vi "SMR_LabVIEW_V8.vi"() -> ()   [LabVIEW 2025]
uses:
  <vilib>/DAQmx/write.llb/DAQmx Write (Analog DBL 1Chan 1Samp).vi
  <vilib>/DAQmx/read.llb/DAQmx Read (Analog 1D DBL NChan 1Samp).vi
  <vilib>/DAQmx/read.llb/DAQmx Read (Analog 2D DBL NChan NSamp).vi
  <vilib>/Analysis/baseanly.llb/Mean (DBL).vi
  <vilib>/DAQmx/create/channels.llb/DAQmx Create Channel (AI-Temperature-Thermocouple).vi
  <vilib>/DAQmx/create/channels.llb/DAQmx Create Channel (AI-Voltage-Basic).vi
  <vilib>/DAQmx/create/channels.llb/DAQmx Create Channel (AO-Voltage-Basic).vi
  <vilib>/DAQmx/miscellaneous.llb/DAQmx Fill In Error Info.vi
  <vilib>/DAQmx/configure/timing.llb/DAQmx Timing (Sample Clock).vi
  <vilib>/addons/control/pid/pid.llb/PID (DBL).vi
  <vilib>/measure/maspectr.llb/FFT Power Spectrum and PSD for 1 Chan.vi
  <vilib>/measure/matone.llb/Extract Single Tone Information 1 Chan.vi
  <vilib>/addons/control/pid/NI_PID_pid.lvlib
  <vilib>/Analysis/NI_AALBase.lvlib
  <vilib>/ptbypt/NI_PtbyPt.lvlib
  <vilib>/measure/NI_MAPro.lvlib
panel:
  out "Time in Steady State (s)":dbl
  in  "Steady-State Dwell (s)":dbl
  out "Main Loop Flow (GPM)":dbl
  out "FM Amplitude":dbl
  out "FM Frequency":dbl
  out "Spectrum":cluster{"f0":dbl, "df":dbl, "magnitude":dbl[]}(graph)
  out "Raw Signal":waveform(dbl)(graph)
  out "Smoothed HX Flow (GPM)":dbl
  out "Flow History":dbl(graph)
  out "HX Flow (GPM)":dbl
  out "Voltage Across Rod (V)":dbl format="%0.2f"
  out "Current Run Folder":path
  in  "Log Root Folder":path=path "C:/Users/LocalUser/Documents/GitHub/thermal-loop/resources/v0.1.1/data/001"
  out "Raw NI9201 \nVoltage Display":T1
  in  "Loop Period (ms)":dbl=1000.0
  in  "Stop":bool
  out "Auto Steady State Threshold (deg C/min)":dbl
  out "Max dT/dt (deg C/min)":dbl
  out "Temp Change Rate (deg C/min)":dbl
  out "5-Min Baseline Complete":bool
  out "Rate Window Ready":bool
  out "Steady State":bool
  in  "Voltage Limit (V)":dbl=10.0
  in  "Temperature Limit (C)":dbl=50.0
  in  "Pressure Limit (psi)":dbl=15.0
  out "Max Voltage":bool
  out "Max Temperature":bool
  out "Max Pressure":bool
  out "Heat Exchanger Pressure History":dbl(graph)
  out "Main Loop Pressure History":T2(graph)
  out "Overall Avg Pressure (psi)":dbl
  out "Heat Exchanger Pressure P6 (psi)":dbl
  out "Main Loop Avg Pressure (psi)":dbl
  out "Pressure Display":T3
  out "Overall Pressure History":T4(graph)
  out "Max Loop Pressure (psi)":dbl
  out "Heat Exchanger Temperature History":cluster{"Waveform":dbl, "Waveform":dbl}(graph)
  out "Main Loop Temeperature History":T5(graph)
  out "Heat Exchanger Avg Temp (deg C)":dbl
  out "Temperature Display":T6
  out "Overall Temperature History":T7(graph)
  out "Overall Avg Temp (deg C)":dbl
  out "Max Loop Temp (deg C)":dbl
  out "Final P-Valve Voltage (V)":dbl
  out "PID Trim Voltage (V)":dbl
  in  "PID Temp Setpoint (deg C)":dbl
  in  "Auto PID Enable":bool
  in  "Manual P-Valve Voltage (V)":dbl min=0.0 max=10.0
  out "Main Loop Avg Temp (deg C)":dbl
  # "Heat Exchanger Flow"
  # "Control/Troubleshoot"
  # "Steady State"
  # "Emergency Indicators"
  # "Pressure"
  # "Temperature"
  # "Proportional Valve Control"
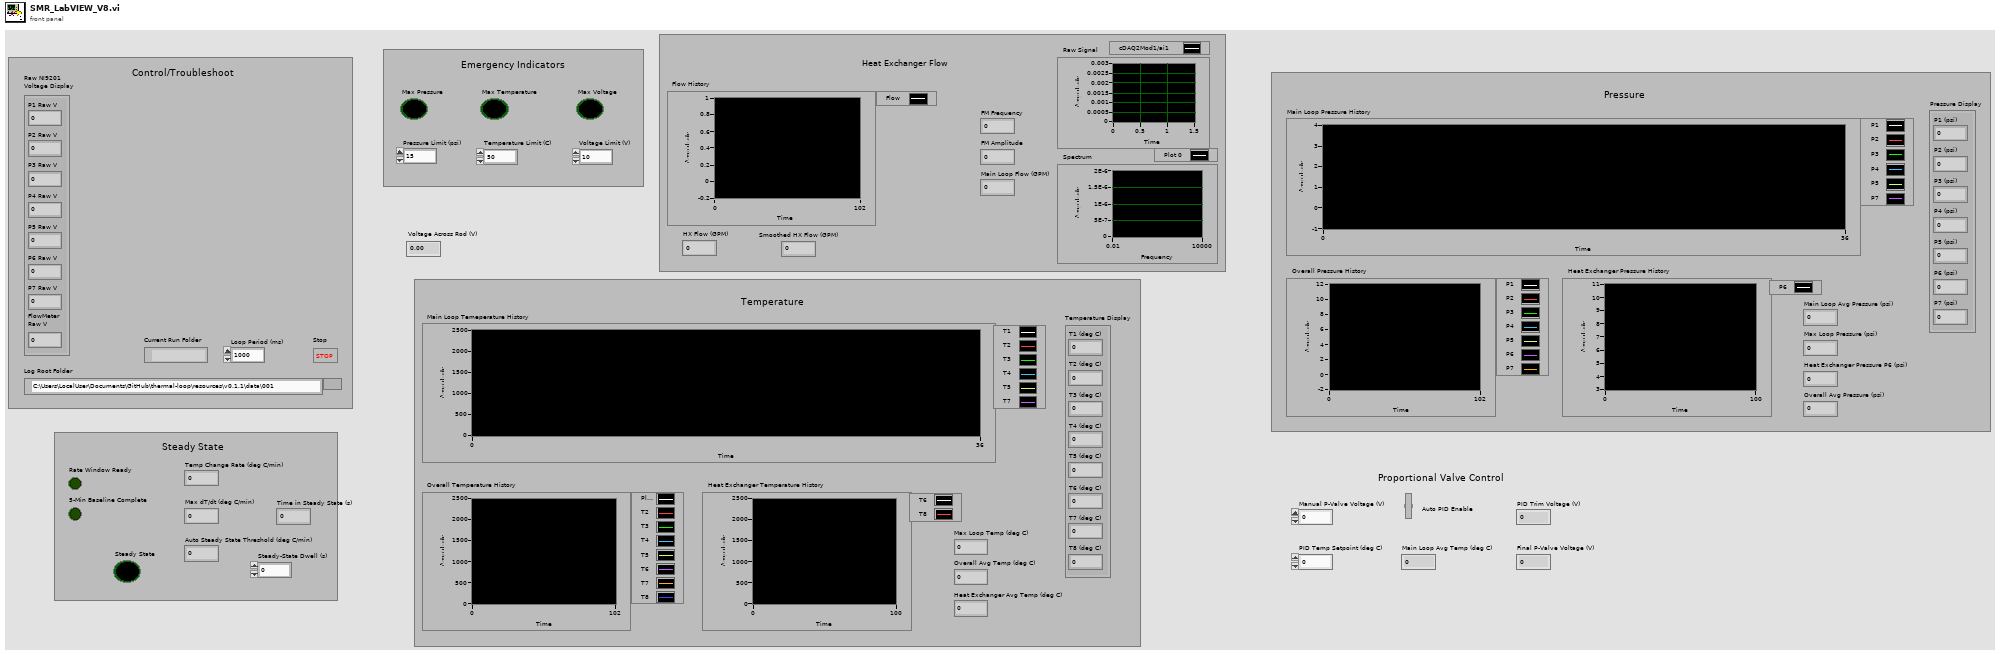
[diagram p1: front panel]
types:
  T1 = cluster{"P1 Raw V":dbl, "P2 Raw V":dbl, "P3 Raw V":dbl, "P4 Raw V":dbl, "P5 Raw V":dbl, "P6 Raw V":dbl, "P7 Raw V":dbl, "FlowMeter\nRaw V":dbl}
  T2 = cluster{"P1":dbl, "P2":dbl, "P3":dbl, "P4":dbl, "P5":dbl, "P7":dbl}
  T3 = cluster{"P1 (psi)":dbl, "P2 (psi)":dbl, "P3 (psi)":dbl, "P4 (psi)":dbl, "P5 (psi)":dbl, "P6 (psi)":dbl, "P7 (psi)":dbl}
  T4 = cluster{"P1":dbl, "P2":dbl, "P3":dbl, "P4":dbl, "P5":dbl, "P6":dbl, "P7":dbl}
  T5 = cluster{"Waveform":dbl, "Waveform":dbl, "Waveform":dbl, "Waveform":dbl, "Waveform":dbl, "Waveform":dbl}
  T6 = cluster{"T1 (deg C)":dbl, "T2 (deg C)":dbl, "T3 (deg C)":dbl, "T4 (deg C)":dbl, "T5 (deg C)":dbl, "T6 (deg C)":dbl, "T7 (deg C)":dbl, "T8 (deg C)":dbl}
  T7 = cluster{"Waveform":dbl, "Waveform":dbl, "Waveform":dbl, "Waveform":dbl, "Waveform":dbl, "Waveform":dbl, "Waveform":dbl, "Waveform":dbl}
  T8 = enum16{"open", "replace", "create", "open or create", "replace or create", "replace or create with confirmation"}
  T9 = cluster{"proportional gain (Kc)":dbl, "integral time (Ti, min)":dbl, "derivative time (Td, min)":dbl}
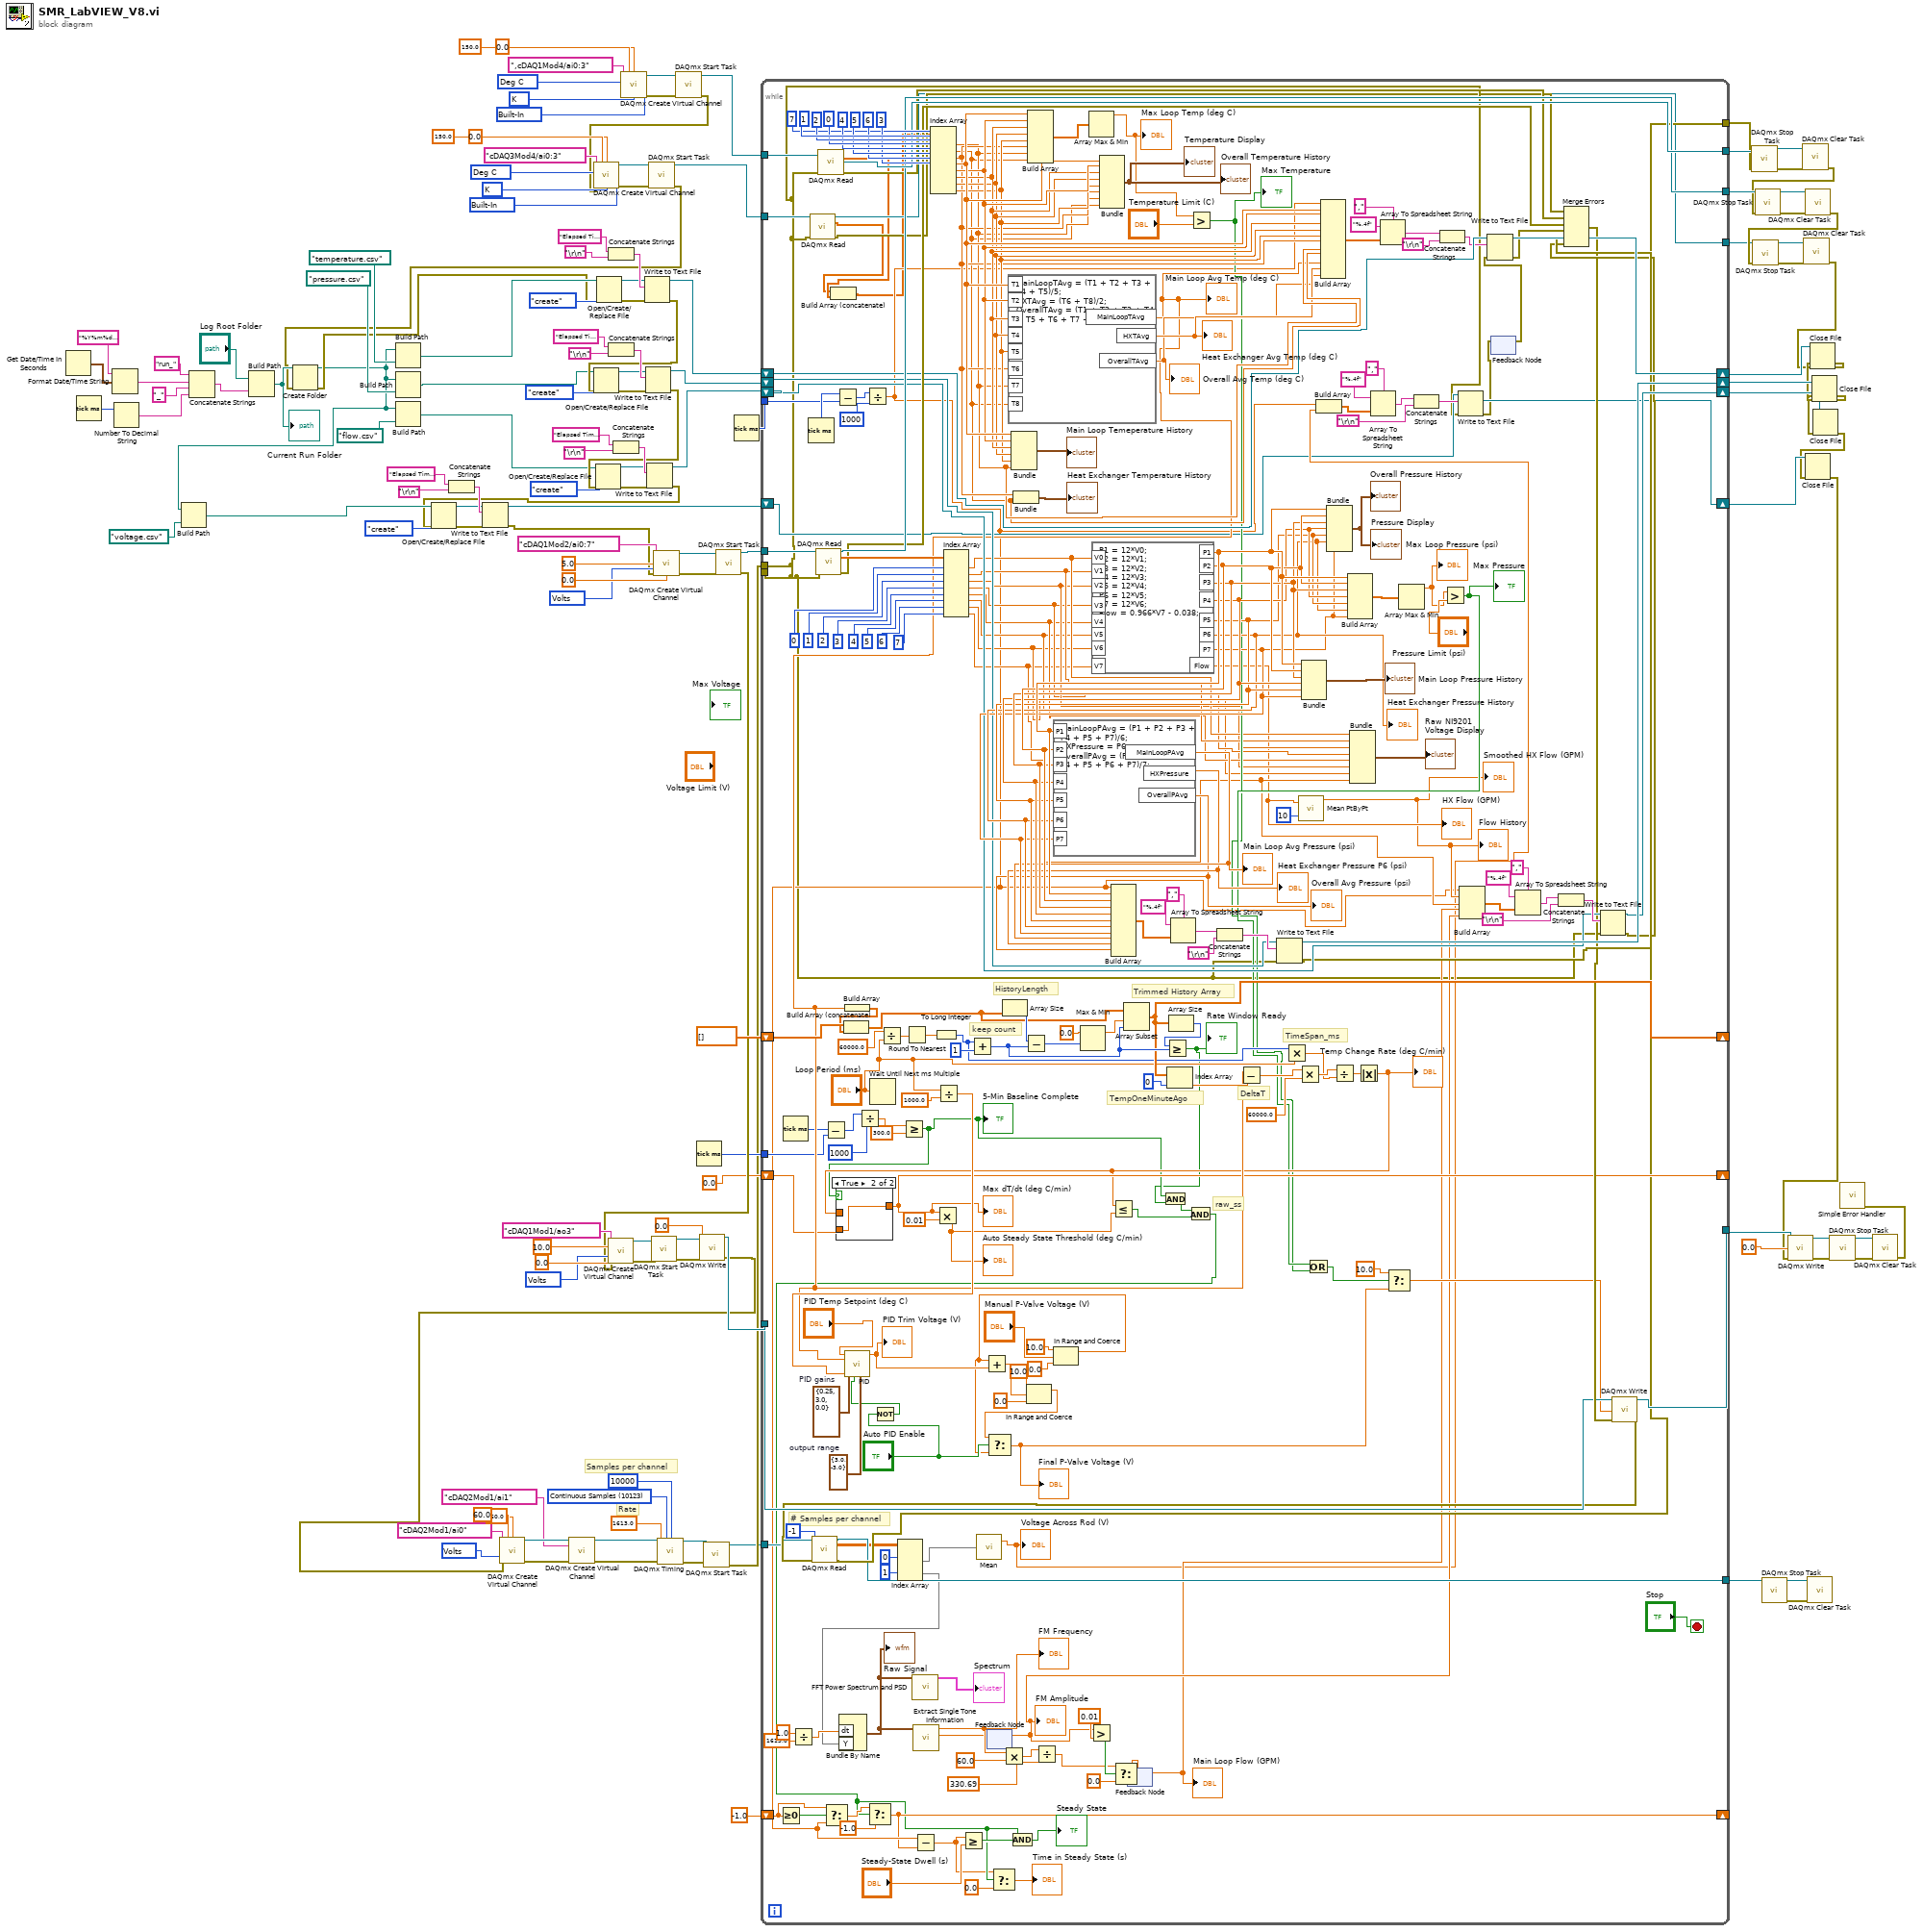
[diagram p0: block diagram]
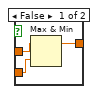
[diagram p2: hidden frame]
diagram:
  w12 = 10200 items=["Built-In"=10200, "Constant Value"=10116, "Channel"=10113] ("cjc source")
  w13 = 10073 items=["J"=10072, "K"=10073, "N"=10077, "R"=10082, "S"=10085, "T"=10086, "B"=10047, "E"=10055] ("thermocouple type")
  w14 = 10143 items=["Deg C"=10143, "Deg F"=10144, "Kelvins"=10325, "Deg R"=10145, "From Custom Scale"=10065] ("units")
  w47 = 10123 items=["Finite Samples"=10178, "Continuous Samples"=10123, "Hardware Timed Single Point"=12522] ("sample mode")
  w49 = 10348 items=["Volts"=10348, "From Custom Scale"=10065] ("units")
  w69 = 10348 items=["Volts"=10348, "From Custom Scale"=10065] ("units")
  w131 = 10200 items=["Built-In"=10200, "Constant Value"=10116, "Channel"=10113] ("cjc source")
  w132 = 10073 items=["J"=10072, "K"=10073, "N"=10077, "R"=10082, "S"=10085, "T"=10086, "B"=10047, "E"=10055] ("thermocouple type")
  w133 = 10143 items=["Deg C"=10143, "Deg F"=10144, "Kelvins"=10325, "Deg R"=10145, "From Custom Scale"=10065] ("units")
  w140 = 10348 items=["Volts"=10348, "From Custom Scale"=10065] ("units")
  # "Samples per channel"
  # "Rate"
  n1 = Get Date/Time In Seconds() -> (seconds since 1Jan1904=w90:timestamp)
  n2 = Tick Count (ms)() -> (millisecond timer value=w88:u32)
  n3 = Format Date/Time String(time format string (%c)="%Y%m%d_%H%M%S", seconds (now)=w90) -> (date/time string=w85:string)  [unwired: 1 in]
  n4 = Number To Decimal String(number=w88) -> (decimal integer string=w86:string)  [unwired: 1 in]
  n5 = Concatenate Strings("run_" ("string"), w85, "_" ("string"), w86) -> (w82:string)
  n6 = Build Path(base path="Log Root Folder", name or relative path=w82) -> (appended path=w81:path)
  "Current Run Folder" <- w81
  n7 = Concatenate Strings("Elapsed Time (s), Rod voltage (V)", "\r\n") -> (w31:string)
  n8 = Concatenate Strings("Elapsed Time (s),T1 (deg C),T2 (deg C),T3 (deg C),T4 (deg C),T5 (deg C),T6 (deg C),T7 (deg C),T8 (deg C),Main Loop Avg Temp (deg C),HX Avg Temp (deg C),Overall Avg Temp (deg C)", "\r\n") -> (w114:string)
  n9 = Concatenate Strings("Elapsed Time (s),P1 (psi),P2 (psi),P3 (psi),P4 (psi),P5 (psi),P6 (psi),P7 (psi),Main Loop Avg Pressure (psi),HX Pressure (psi),Overall Avg Pressure (psi)", "\r\n") -> (w112:string)
  n10 = Concatenate Strings("Elapsed Time (s),Heat Exchanger Flow (GPM),Flow Raw Voltage (V), Main Loop Flow (GPM), Flow Signal Amplitude (V)", "\r\n") -> (w108:string)
  n11 = call-poly <vilib>:"DAQmx Create Virtual Channel.vi"("maximum value"=150.0, "minimum value"=0.0, "physical channels"=tag ",cDAQ1Mod4/ai0:3", "cjc source"=w131, "units"=w133, "thermocouple type"=w132) -> ("task out"=w130:refnum<k21>, "error out"=w129:errorcluster)  [unwired: 8 in]
  n12 = call <vilib>:"DAQmx Start Task.vi"("task/channels in"=w130, "error in"=w129) -> ("task out"=w128:refnum<k21>, "error out"=w8:errorcluster)  [unwired: 12 in]
  n13 = call-poly <vilib>:"DAQmx Create Virtual Channel.vi"("maximum value"=150.0, "minimum value"=0.0, "physical channels"=tag "cDAQ3Mod4/ai0:3", "cjc source"=w12, "units"=w14, "error in"=w8, "thermocouple type"=w13) -> ("task out"=w11:refnum<k21>, "error out"=w10:errorcluster)  [unwired: 7 in]
  n14 = call <vilib>:"DAQmx Start Task.vi"("task/channels in"=w11, "error in"=w10) -> ("task out"=w6:refnum<k21>, "error out"=w7:errorcluster)  [unwired: 12 in]
  n15 = Create Folder(path (use dialog)=w81, error in=w7) -> (created path=w25:path, error out=w74:errorcluster)  [unwired: 1 in, 1 out]
  n16 = Build Path(base path=w25, name or relative path=path "voltage.csv") -> (appended path=w26:path)
  n17 = Build Path(base path=w25, name or relative path=path "temperature.csv") -> (appended path=w80:path)
  n18 = Build Path(base path=w25, name or relative path=path "pressure.csv") -> (appended path=w79:path)
  n19 = Build Path(base path=w25, name or relative path=path "flow.csv") -> (appended path=w78:path)
  n20 = Open/Create/Replace File(file path (use dialog)=w80, error in=w74, operation (0:open)=T8."create") -> (refnum out=w113:refnum<file>, error out=w97:errorcluster)  [unwired: 3 in, 1 out]
  n21 = Write to Text File(file (use dialog)=w113, text=w114, error in=w97) -> (refnum out=w104:refnum<file>, error out=w96:errorcluster)  [unwired: 1 in, 1 out]
  n22 = Open/Create/Replace File(file path (use dialog)=w79, error in=w96, operation (0:open)=T8."create") -> (refnum out=w111:refnum<file>, error out=w95:errorcluster)  [unwired: 3 in, 1 out]
  n23 = Write to Text File(file (use dialog)=w111, text=w112, error in=w95) -> (refnum out=w103:refnum<file>, error out=w94:errorcluster)  [unwired: 1 in, 1 out]
  n24 = Open/Create/Replace File(file path (use dialog)=w78, error in=w94, operation (0:open)=T8."create") -> (refnum out=w107:refnum<file>, error out=w93:errorcluster)  [unwired: 3 in, 1 out]
  n25 = Write to Text File(file (use dialog)=w107, text=w108, error in=w93) -> (refnum out=w102:refnum<file>, error out=w23:errorcluster)  [unwired: 1 in, 1 out]
  n26 = Open/Create/Replace File(file path (use dialog)=w26, error in=w23, operation (0:open)=T8."create") -> (refnum out=w30:refnum<file>, error out=w27:errorcluster)  [unwired: 3 in, 1 out]
  n27 = Write to Text File(file (use dialog)=w30, text=w31, error in=w27) -> (refnum out=w21:refnum<file>, error out=w22:errorcluster)  [unwired: 1 in, 1 out]
  n28 = call-poly <vilib>:"DAQmx Create Virtual Channel.vi"("maximum value"=5.0, "minimum value"=0.0, "physical channels"=tag "cDAQ1Mod2/ai0:7", "units"=w140, "error in"=w22) -> ("task out"=w139:refnum<k21>, "error out"=w138:errorcluster)  [unwired: 9 in]
  n29 = Tick Count (ms)() -> (millisecond timer value=w54:u32)
  n30 = call <vilib>:"DAQmx Start Task.vi"("task/channels in"=w139, "error in"=w138) -> ("task out"=w137:refnum<k21>, "error out"=w62:errorcluster)  [unwired: 12 in]
  n31 = call-poly <vilib>:"DAQmx Create Virtual Channel.vi"("maximum value"=10.0, "minimum value"=0.0, "physical channels"=tag "cDAQ1Mod1/ao3", "units"=w69, "error in"=w62) -> ("task out"=w68:refnum<k21>, "error out"=w67:errorcluster)  [unwired: 9 in]
  n32 = call <vilib>:"DAQmx Start Task.vi"("task/channels in"=w68, "error in"=w67) -> ("task out"=w66:refnum<k21>, "error out"=w65:errorcluster)  [unwired: 12 in]
  n33 = call-poly <vilib>:"DAQmx Write.vi"("task/channels in"=w66, "data"=0.0, "error in"=w65) -> ("task out"=w63:refnum<k21>, "error out"=w41:errorcluster)  [unwired: 10 in, 1 out]
  n34 = call-poly <vilib>:"DAQmx Create Virtual Channel.vi"("maximum value"=60.0, "minimum value"=-60.0, "physical channels"=tag "cDAQ2Mod1/ai0", "units"=w49, "error in"=w41) -> ("task out"=w37:refnum<k21>, "error out"=w36:errorcluster)  [unwired: 9 in]
  n35 = call-poly <vilib>:"DAQmx Create Virtual Channel.vi"("task in"=w37, "physical channels"=tag "cDAQ2Mod1/ai1", "error in"=w36) -> ("task out"=w35:refnum<k21>, "error out"=w34:errorcluster)  [unwired: 11 in]
  n36 = call-poly <vilib>:"DAQmx Timing.vi"("task/channels in"=w35, "sample mode"=w47, "samples per channel"=10000, "rate"=1613.0, "error in"=w34) -> ("task out"=w45:refnum<k21>, "error out"=w44:errorcluster)  [unwired: 9 in]
  n37 = call <vilib>:"DAQmx Start Task.vi"("task/channels in"=w45, "error in"=w44) -> ("task out"=w39:refnum<k21>, "error out"=w40:errorcluster)  [unwired: 12 in]
  n38 = Tick Count (ms)() -> (millisecond timer value=w101:u32)
  n39 = while {
    tunnel: w137 -> [w361]
    tunnel: w128 -> [w344]
    tunnel: [w335] -> w127
    tunnel: [w149] -> _
    tunnel: [w334] -> w126
    tunnel: [w210] -> w125
    shift-right: [w311] -> w100
    shift-left: w104 -> [w312]
    shift-right: [w292] -> w99
    shift-left: w103 -> [w293]
    shift-right: [w284] -> w98
    shift-left: w102 -> [w285]
    tunnel: w101 -> [w330]
    shift-right: [w263] -> _
    shift-left: dbl[] [] -> [w276]
    tunnel: w63 -> [w244]
    tunnel: w40 -> [w149]
    tunnel: [w251] -> w60
    tunnel: w54 -> [w233]
    shift-right: [w226] -> _
    shift-left: 0.0 -> [w228]
    tunnel: w39 -> [w209]
    tunnel: [w208] -> w38
    shift-right: [w166] -> w20
    shift-left: w21 -> [w167]
    shift-right: [w158] -> _
    shift-left: -1.0 -> [w162]
    tunnel: w6 -> [w150]
    tunnel: [w147] -> w2
    stop <- "Stop" stop-if-true
    w249 = cluster{"output high":dbl, "output low":dbl} {"output high"=3.0, "output low"=-3.0}  # output range
    w250 = T9 {"proportional gain (Kc)"=0.25, "integral time (Ti, min)"=3.0, "derivative time (Td, min)"=0.0}  # PID gains
    # "raw_ss"
    # "# Samples per channel"
    # "TimeSpan_ms"
    # "DeltaT"
    # "TempOneMinuteAgo"
    # "Trimmed History Array"
    # "HistoryLength"
    # "keep count"
    n40 = Greater Or Equal To 0?(x=w162) -> (x >= 0?=w163:bool)
    n41 = Tick Count (ms)() -> (millisecond timer value=w234:u32)
    n42 = Divide(x=1.0, y=1613.0) -> (x/y=w181:dbl)
    n43 = Tick Count (ms)() -> (millisecond timer value=w331:u32)
    n44 = call-poly <vilib>:"DAQmx Read.vi"("task/channels in"=w150, "error in"=w149) -> ("task out"=w147:refnum<k21>, "data"=w144:dbl[], "error out"=w148:errorcluster)  [unwired: 11 in]
    n45 = call-poly <vilib>:"DAQmx Read.vi"("task/channels in"=w361, "error in"=w149) -> ("task out"=w334:refnum<k21>, "data"=w352:dbl[], "error out"=w332:errorcluster)  [unwired: 11 in]
    n46 = call-poly <vilib>:"DAQmx Read.vi"("task/channels in"=w344, "error in"=w149) -> ("task out"=w335:refnum<k21>, "data"=w145:dbl[], "error out"=w333:errorcluster)  [unwired: 11 in]
    n47 = Subtract(x=w234, y=w233) -> (x-y=w232:u32)
    n48 = Build Array (concatenate)(w144, w145) -> (w146:dbl[])
    n49 = Subtract(x=w331, y=w330) -> (x-y=w329:u32)
    n50 = Divide(x=w232, y=u32 1000) -> (x/y=w230:dbl)
    n51 = Divide(x=w329, y=u32 1000) -> (x/y=w159:dbl)
    n52 = Select(t=w162, s=w163, f=w159) -> (s? t:f=w161:dbl)
    n53 = Wait Until Next ms Multiple(millisecond multiple="Loop Period (ms)") -> ()  [unwired: 1 out]
    n54 = Not(x="Auto PID Enable") -> (.not. x?=w245:bool)
    n55 = Divide(x=60000.0, y="Loop Period (ms)") -> (x/y=w273:dbl)
    n56 = Greater Or Equal?(x=w230, y=300.0) -> (x >= y?=w223:bool)
    "5-Min Baseline Complete" <- w223
    n57 = Round To Nearest(number=w273) -> (nearest integer value=w272:dbl)
    n58 = Index Array(array=w146, index #1=7 ("index"), index #2=1 ("index"), index #3=2 ("index"), index #4=0 ("index"), index #5=4 ("index"), index #6=5 ("index"), index #7=6 ("index"), index #8=3 ("index")) -> (element #1=w321:dbl, element #2=w320:dbl, element #3=w322:dbl, element #4=w327:dbl, element #5=w326:dbl, element #6=w325:dbl, element #7=w324:dbl, element #8=w323:dbl)
    n59 = To Long Integer(number=w272) -> (32bit integer=w260:i32)
    n60 = Divide(x="Loop Period (ms)", y=1000.0) -> (x/y=w246:dbl)
    n61 = Index Array(array=w352, index #1=0 ("index"), index #2=1 ("index"), index #3=2 ("index"), index #4=3 ("index"), index #5=4 ("index"), index #6=5 ("index"), index #7=6 ("index"), index #8=7 ("index")) -> (element #1=w207:dbl, element #2=w206:dbl, element #3=w205:dbl, element #4=w204:dbl, element #5=w203:dbl, element #6=w202:dbl, element #7=w201:dbl, element #8=w200:dbl)
    n62 = Add(x=w260, y=1) -> (x+y=w265:i32)
    n63 = feedback #1() -> (w177:dbl)  [unwired: 1 in]
    "FM Amplitude" <- w177
    n64 = formula code="MainLoopTAvg = (T1 + T2 + T3 + T4 + T5)/5;\nHXTAvg = (T6 + T8)/2;\nOverallTAvg = (T1 + T2 + T3 + T4 + T5 + T6 + T7 + T8)/8;"("T1"=w327, "T2"=w326, "T3"=w325, "T4"=w324, "T5"=w323, "T6"=w322, "T7"=w321, "T8"=w320) -> ("MainLoopTAvg"=w236:dbl, "HXTAvg"=w319:dbl, "OverallTAvg"=w318:dbl)
    "Overall Avg Temp (deg C)" <- w318
    "Main Loop Avg Temp (deg C)" <- w236
    "Heat Exchanger Avg Temp (deg C)" <- w319
    n65 = Build Array(w236) -> (w275:dbl[])
    n66 = Build Array (concatenate)(w276, w275) -> (w267:dbl[])
    n67 = call-poly <vilib>:"PID.vi"("reinitialize? (F)"=w245, "output range"=w249, "dt (s)"=w246, "PID gains"=w250, "process variable"=w236, "setpoint"="PID Temp Setpoint (deg C)") -> ("output"=w243:dbl)  [unwired: 4 in, 1 out]
    "PID Trim Voltage (V)" <- w243
    n68 = Array Size(array=w267) -> (size(s)=w270:i32)
    n69 = Bundle("Waveform"=w327, "Waveform"=w326, "Waveform"=w325, "Waveform"=w324, "Waveform"=w323, "Waveform"=w321) -> (→"Main Loop Temeperature History":T5)  [unwired: 1 in]
    n70 = Bundle("Waveform"=w322, "Waveform"=w320) -> (→"Heat Exchanger Temperature History":cluster{"Waveform":dbl, "Waveform":dbl})  [unwired: 1 in]
    n71 = Subtract(x=w270, y=w265) -> (x-y=w268:i32)
    n72 = Build Array(w327, w326, w325, w324, w323, w322, w321, w320) -> (w362:dbl[])
    n73 = In Range and Coerce(upper limit=10.0, x="Manual P-Valve Voltage (V)", lower limit=0.0) -> (coerced(x)=w238:dbl)  [unwired: 1 out]
    n74 = Add(x=w238, y=w243) -> (x+y=w242:dbl)
    n75 = In Range and Coerce(upper limit=10.0, x=w242, lower limit=0.0) -> (coerced(x)=w237:dbl)  [unwired: 1 out]
    n76 = Select(t=w237, s="Auto PID Enable", f=w238) -> (s? t:f=w215:dbl)
    "Final P-Valve Voltage (V)" <- w215
    n77 = Max & Min(x=0.0, y=w268) -> (max(x,y)=w266:dbl)  [unwired: 1 out]
    n78 = Array Max & Min(array=w362) -> (max value=w278:dbl)  [unwired: 3 out]
    "Max Loop Temp (deg C)" <- w278
    n79 = Greater?(x=w177, y=0.01) -> (0:w185:bool)
    n80 = formula code="P1 = 12*V0;\nP2 = 12*V1;\nP3 = 12*V2;\nP4 = 12*V3;\nP5 = 12*V4;\nP6 = 12*V5; \nP7 = 12*V6;\nFlow = 0.966*V7 - 0.038;"("V0"=w207, "V1"=w206, "V2"=w205, "V3"=w204, "V4"=w203, "V5"=w202, "V6"=w201, "V7"=w200) -> ("P1"=w310:dbl, "P2"=w309:dbl, "P3"=w308:dbl, "P4"=w307:dbl, "P5"=w306:dbl, "P6"=w305:dbl, "P7"=w304:dbl, "Flow"=w199:dbl)
    "HX Flow (GPM)" <- w199
    "Heat Exchanger Pressure History" <- w305
    n81 = formula code="MainLoopPAvg = (P1 + P2 + P3 + P4 + P5 + P7)/6;\nHXPressure = P6;\nOverallPAvg = (P1 + P2 + P3 + P4 + P5 + P6 + P7)/7;"("P1"=w310, "P2"=w309, "P3"=w308, "P4"=w307, "P5"=w306, "P6"=w305, "P7"=w304) -> ("MainLoopPAvg"=w303:dbl, "HXPressure"=w302:dbl, "OverallPAvg"=w301:dbl)
    "Overall Avg Pressure (psi)" <- w301
    "Heat Exchanger Pressure P6 (psi)" <- w302
    "Main Loop Avg Pressure (psi)" <- w303
    n82 = Bundle("Waveform"=w327, "Waveform"=w326, "Waveform"=w325, "Waveform"=w324, "Waveform"=w323, "Waveform"=w322, "Waveform"=w321, "Waveform"=w320) -> (→"Overall Temperature History" →"Temperature Display":T7)  [unwired: 1 in]
    n83 = Build Array(w159, w310, w309, w308, w307, w306, w305, w304, w303, w302, w301) -> (w300:dbl[])
    n84 = Array Subset(array=w267, index=w266, length=w265) -> (w263:dbl[])
    n85 = feedback #2() -> (w175:dbl)  [unwired: 1 in]
    "Main Loop Flow (GPM)" <- w175
    n86 = Index Array(array=w263, index=0) -> (element=w261:dbl)
    n87 = Array Size(array=w263) -> (size(s)=w264:i32)
    n88 = Greater Or Equal?(x=w264, y=w265) -> (x >= y?=w222:bool)
    "Rate Window Ready" <- w222
    n89 = And(x=w223, y=w222) -> (x .and. y?=w221:bool)
    n90 = Array To Spreadsheet String(delimiter (Tab)=",", array=w300, 3:"%.4f" ("format string")) -> (spreadsheet string=w296:string)
    n91 = Greater?(x=w278, y="Temperature Limit (C)") -> (0:w218:bool)
    "Max Temperature" <- w218
    n92 = Concatenate Strings(w296, "\r\n") -> (w294:string)
    n93 = Subtract(x=w236, y=w261) -> (x-y=w259:dbl)
    n94 = Write to Text File(file (use dialog)=w293, text=w294, error in=w149) -> (refnum out=w292:refnum<file>, error out=w282:errorcluster)  [unwired: 1 in, 1 out]
    n95 = Multiply(x=w260, y="Loop Period (ms)") -> (x*y=w256:dbl)
    n96 = Multiply(x=w259, y=60000.0) -> (x*y=w257:dbl)
    n97 = call <vilib>:"Mean PtByPt.vi"("x"=w199, "sample length"=10) -> ("mean"=w197:dbl)  [unwired: 2 in, 1 out]
    "Flow History" <- w197
    "Smoothed HX Flow (GPM)" <- w197
    n98 = Bundle("P1"=w310, "P2"=w309, "P3"=w308, "P4"=w307, "P5"=w306, "P7"=w304) -> (→"Main Loop Pressure History":T2)  [unwired: 1 in]
    n99 = Build Array(w159, w327, w326, w325, w324, w323, w322, w321, w320, w236, w319, w318) -> (w317:dbl[])
    n100 = Bundle("P1"=w310, "P2"=w309, "P3"=w308, "P4"=w307, "P5"=w306, "P6"=w305, "P7"=w304) -> (→"Overall Pressure History" →"Pressure Display":T4)  [unwired: 1 in]
    n101 = Divide(x=w257, y=w256) -> (x/y=w255:dbl)
    n102 = Build Array(w310, w309, w308, w307, w306, w305, w304) -> (w351:dbl[])
    n103 = Bundle("Waveform"=w207, "Waveform"=w206, "Waveform"=w205, "Waveform"=w204, "Waveform"=w203, "Waveform"=w202, "Waveform"=w201, "Waveform"=w200) -> (→"Raw NI9201 \nVoltage Display":T7)  [unwired: 1 in]
    n104 = Absolute Value(x=w255) -> (abs(x)=w225:dbl)
    "Temp Change Rate (deg C/min)" <- w225
    n105 = case shown="True" w223 {
      tunnel: w228 -> [w366 w367]
      tunnel: w225 -> [w365 _]
      tunnel: [w364 w367] -> w226
      frame False {
        n106 = Max & Min(x=w365, y=w366) -> (max(x,y)=w364:dbl)  [unwired: 1 out]
      }
      frame True {
      }
    }
    "Max dT/dt (deg C/min)" <- w226
    n107 = Multiply(x=w226, y=0.01) -> (x*y=w224:dbl)
    "Auto Steady State Threshold (deg C/min)" <- w224
    n108 = Less Or Equal?(x=w225, y=w224) -> (x <= y?=w220:bool)
    n109 = And(x=w221, y=w220) -> (x .and. y?=w154:bool)
    n110 = Select(t=w161, s=w154, f=-1.0) -> (s? t:f=w158:dbl)
    n111 = Subtract(x=w159, y=w158) -> (x-y=w153:dbl)
    n112 = Greater Or Equal?(x=w153, y="Steady-State Dwell (s)") -> (x >= y?=w156:bool)
    n113 = Select(t=w153, s=w154, f=0.0) -> (s? t:f=→"Time in Steady State (s)":dbl)
    n114 = And(x=w154, y=w156) -> (x .and. y?=→"Steady State":bool)
    n115 = Array To Spreadsheet String(delimiter (Tab)=",", array=w317, 3:"%.4f" ("format string")) -> (spreadsheet string=w314:string)
    n116 = Array Max & Min(array=w351) -> (max value=w279:dbl)  [unwired: 3 out]
    "Max Loop Pressure (psi)" <- w279
    n117 = Concatenate Strings(w314, "\r\n") -> (w297:string)
    n118 = Greater?(x=w279, y="Pressure Limit (psi)") -> (0:w219:bool)
    "Max Pressure" <- w219
    n119 = Or(x=w219, y=w218) -> (x .or. y?=w213:bool)
    n120 = Select(t=10.0, s=w213, f=w215) -> (s? t:f=w214:dbl)
    n121 = Build Array(w159, w197, w200, w175, w177) -> (w291:dbl[])
    n122 = feedback #3() -> (w164:errorcluster)  [unwired: 1 in]
    n123 = Write to Text File(file (use dialog)=w312, text=w297, error in=w164) -> (refnum out=w311:refnum<file>, error out=w283:errorcluster)  [unwired: 1 in, 1 out]
    n124 = Array To Spreadsheet String(delimiter (Tab)=",", array=w291, 3:"%.4f" ("format string")) -> (spreadsheet string=w287:string)
    n125 = Concatenate Strings(w287, "\r\n") -> (w286:string)
    n126 = Write to Text File(file (use dialog)=w285, text=w286, error in=w149) -> (refnum out=w284:refnum<file>, error out=w281:errorcluster)  [unwired: 1 in, 1 out]
    n127 = Merge Errors(w148, w333, w332, w283, w282, w281) -> (w252:errorcluster)
    n128 = call-poly <vilib>:"DAQmx Write.vi"("task/channels in"=w244, "data"=w214, "error in"=w252) -> ("task out"=w251:refnum<k21>, "error out"=w211:errorcluster)  [unwired: 10 in, 1 out]
    n129 = call-poly <vilib>:"DAQmx Read.vi"("task/channels in"=w209, "number of samples per channel"=-1, "error in"=w211) -> ("task out"=w208:refnum<k21>, "data"=w196:dbl[][], "error out"=w210:errorcluster)  [unwired: 10 in]
    n130 = Index Array(array=w196, index (row) #1=0 ("index (row)"), index (row) #2=1 ("index (row)")) -> (element #1=w195:dbl[], element #2=w180:dbl[])  [unwired: 2 in]
    n131 = Bundle By Name("dt"=w181, "Y"=w180) -> (w179:waveform(dbl))  [unwired: 1 in]
    "Raw Signal" <- w179
    n132 = call-poly <vilib>:"FFT Power Spectrum and PSD.vi"("time signal"=w179) -> ("Power Spectrum / PSD"=→"Spectrum":cluster{"f0":dbl, "df":dbl, "magnitude":dbl[]})  [unwired: 7 in, 3 out]
    n133 = call-poly <vilib>:"Extract Single Tone Information.vi"("time signal in"=w179) -> ("detected amplitude"=w178:dbl, "detected frequency"=w191:dbl)  [unwired: 5 in, 4 out]
    "FM Frequency" <- w191
    n134 = call-poly <vilib>:"Mean.vi"("X"=w195) -> ("mean"=w170:dbl)  [unwired: 1 out]
    "Voltage Across Rod (V)" <- w170
    n135 = feedback-in #1(w178) -> ()
    n136 = Multiply(x=w191, y=60.0) -> (x*y=w189:dbl)
    n137 = Divide(x=w189, y=330.69) -> (x/y=w184:dbl)
    n138 = Select(t=w184, s=w185, f=0.0) -> (s? t:f=w176:dbl)
    n139 = feedback-in #2(w176) -> ()
    n140 = Build Array(w159, w170) -> (w169:dbl[])
    n141 = Array To Spreadsheet String(delimiter (Tab)=",", array=w169, 3:"%.4f" ("format string")) -> (spreadsheet string=w173:string)
    n142 = Concatenate Strings(w173, "\r\n") -> (w168:string)
    n143 = Write to Text File(file (use dialog)=w167, text=w168, error in=w149) -> (refnum out=w166:refnum<file>, error out=w165:errorcluster)  [unwired: 1 in, 1 out]
    n144 = feedback-in #3(w165) -> ()
  }
  n145 = call <vilib>:"DAQmx Stop Task.vi"("task/channels in"=w127, "error in"=w125) -> ("task out"=w124:refnum<k21>, "error out"=w122:errorcluster)  [unwired: 12 in]
  n146 = call <vilib>:"DAQmx Stop Task.vi"("task/channels in"=w38) -> ("task out"=w43:refnum<k21>, "error out"=w42:errorcluster)  [unwired: 13 in]
  n147 = call <vilib>:"DAQmx Clear Task.vi"("task in"=w124, "error in"=w122) -> ("error out"=w121:errorcluster)  [unwired: 13 in]
  n148 = call <vilib>:"DAQmx Stop Task.vi"("task/channels in"=w126, "error in"=w121) -> ("task out"=w123:refnum<k21>, "error out"=w120:errorcluster)  [unwired: 12 in]
  n149 = call <vilib>:"DAQmx Clear Task.vi"("task in"=w123, "error in"=w120) -> ("error out"=w5:errorcluster)  [unwired: 13 in]
  n150 = call <vilib>:"DAQmx Stop Task.vi"("task/channels in"=w2, "error in"=w5) -> ("task out"=w1:refnum<k21>, "error out"=w4:errorcluster)  [unwired: 12 in]
  n151 = call <vilib>:"DAQmx Clear Task.vi"("task in"=w1, "error in"=w4) -> ("error out"=w3:errorcluster)  [unwired: 13 in]
  n152 = call <vilib>:"DAQmx Clear Task.vi"("task in"=w43, "error in"=w42) -> ()  [unwired: 13 in, 1 out]
  n153 = Close File(refnum=w100, error in=w3) -> (error out=w92:errorcluster)  [unwired: 1 out]
  n154 = Close File(refnum=w99, error in=w92) -> (error out=w91:errorcluster)  [unwired: 1 out]
  n155 = Close File(refnum=w98, error in=w91) -> (error out=w19:errorcluster)  [unwired: 1 out]
  n156 = Close File(refnum=w20, error in=w19) -> (error out=w18:errorcluster)  [unwired: 1 out]
  n157 = call-poly <vilib>:"DAQmx Write.vi"("task/channels in"=w60, "data"=0.0, "error in"=w18) -> ("task out"=w59:refnum<k21>, "error out"=w57:errorcluster)  [unwired: 10 in, 1 out]
  n158 = call <vilib>:"DAQmx Stop Task.vi"("task/channels in"=w59, "error in"=w57) -> ("task out"=w58:refnum<k21>, "error out"=w56:errorcluster)  [unwired: 12 in]
  n159 = call <vilib>:"DAQmx Clear Task.vi"("task in"=w58, "error in"=w56) -> ("error out"=w55:errorcluster)  [unwired: 13 in]
  n160 = call <vilib>:"Simple Error Handler.vi"("error in (no error)"=w55) -> ()  [unwired: 4 in, 5 out]
